vi "DataLog Tag and Meta Live_srv.vi"(0 "initial?":bool, 5 "read indices in":i32[](array[numeric]), 7 "certificate":string, 11 "base tag":string) -> (6 "read indices out":i32[](array[numeric]), 8 "points per tag":cluster{T1[]}[](array[cluster]) {"?"."value" format="%.3e"; "?"."time" format="%<%H:%M:%S%2u\n%Y/%m/%d>T"}, 10 "time":dbl format="%<%H:%M:%S%2u\n%Y/%m/%d>T", 15 "error out":errorcluster)   [LabVIEW 2012]
doc: "Reads all (when initial is true) or newer (when initial is false) data points from the in-memory buffers of a subset of tags. The read indices beyond the last read point are also returned. This allows a remote exhaustive read of multiple tags using a single VI server call thereby minimizing network load and latency."
uses:
  typedefs/clusters/t_DataLog Point.ctl
  typedefs/t_DataLog Tag Meta Tags Methods.ctl
  typedefs/t_DataLog Tag Hash Methods.ctl
  clientsrv/typedefs/t_ClientSrv Access Levels.ctl
  typedefs/t_DataLog Tag Buffers Methods.ctl
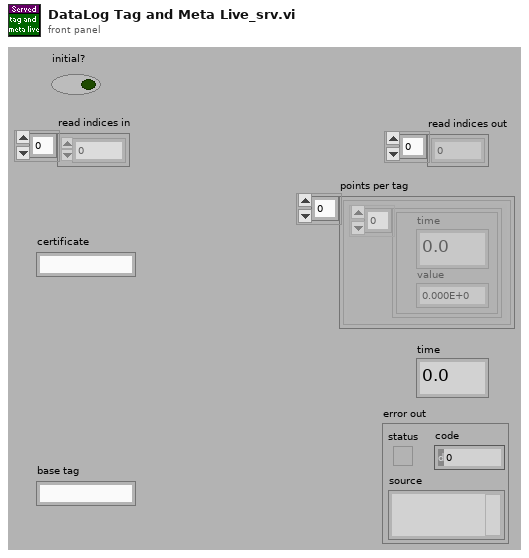
[diagram p1: front panel]
types:
  T1 = typedef "t_DataLog Point.ctl" = cluster{"time":dbl, "value":dbl}
  T2 = typedef "t_ClientSrv Access Levels.ctl" = enum16{"observer", "operator", "local"}
  T3 = typedef "t_DataLog Tag Hash Methods.ctl" = enum16{"initialize", "add tag", "index tag", "lookup", "#tags", "cleanup", "write recovery", "read recovery", "delete recovery"}
  T4 = typedef "t_DataLog Tag Meta Tags Methods.ctl" = enum16{"initialize", "apply and write", "get exceeded", "get metas", "cleanup"}
  T5 = typedef "t_DataLog Tag Buffers Methods.ctl" = enum16{"initialize", "inert", "write", "read", "read oldest", "read last", "cleanup"}
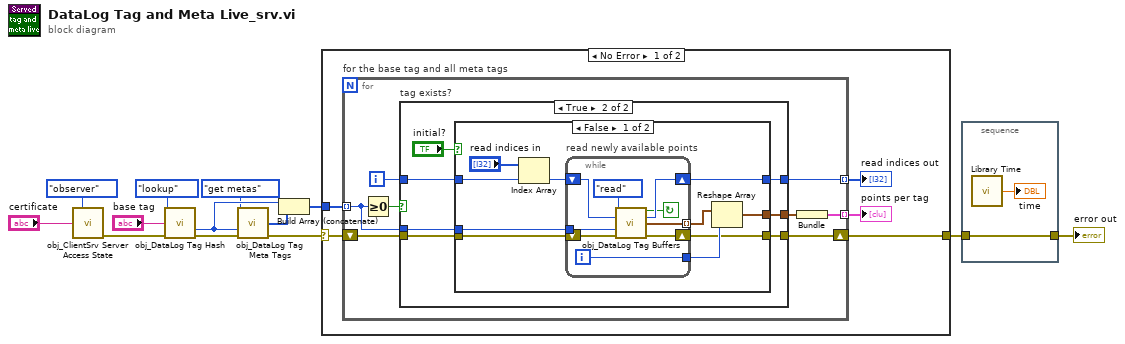
[diagram p0: block diagram]
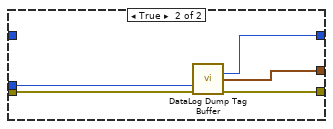
[diagram p3: hidden frame]
diagram:
  n1 = call "obj_ClientSrv Server Access State.vi"("access level"=t_ClientSrv_Access_Levels."observer", "certificate in"="certificate") -> ("error out"=w3:errorcluster)  [unwired: 11 in, 2 out]
  n2 = call "obj_DataLog Tag Hash.vi"("method"=t_DataLog_Tag_Hash_Methods."lookup", "tag in"="base tag", "error in (no error)"=w3) -> ("tag index out"=w12:i32, "error out"=w8:errorcluster)  [unwired: 9 in, 2 out]
  n3 = call "obj_DataLog Tag Meta Tags.vi"("method"=t_DataLog_Tag_Meta_Tags_Methods."get metas", "tag index in"=w12, "error in (no error)"=w8) -> ("meta tag indices (-1 if none)"=w13:i32[], "error out"=w6:errorcluster)  [unwired: 8 in, 3 out]
  n4 = Build Array (concatenate)(w12, w13) -> (w7:i32[])
  n5 = case shown="No Error" w6 {
    selector: w6 -> [w17 w59]
    tunnel: w7 -> [w18 _]
    tunnel: [w16 w59] -> w5
    frame No Error {
      n6 = for "for the base tag and all meta tags" {
        tunnel: w18 -> [w25] mode=indexing
        shift-right: [w23] -> w16
        shift-left: w17 -> [w24]
        tunnel: [w21] -> w15 mode=indexing
        tunnel: [w20] -> w14 mode=indexing
        i -> [w19]
        n7 = Greater Or Equal To 0?(x=w25) -> (x >= 0?=w26:bool)
        n8 = case "tag exists?" shown="True" w26 {
          tunnel: w25 -> [_ w29]
          tunnel: w24 -> [w27 w33]
          tunnel: [w27 w32] -> w23
          tunnel: [_ w31] -> w22
          tunnel: [_ w30] -> w20
          tunnel: w19 -> [_ w28]
          frame False {
          }
          frame True {
            n9 = case shown="False" "initial?" {
              tunnel: w33 -> [w44 w58]
              tunnel: [w38 w57] -> w32
              tunnel: [w40 w56] -> w31
              tunnel: [w42 w54] -> w30
              tunnel: w29 -> [w43 w55]
              tunnel: w28 -> [w35 _]
              frame False {
                n10 = Index Array(array="read indices in", index=w35) -> (element=w37:i32)
                n11 = while "read newly available points" {
                  shift-right: [w52] -> w38
                  shift-left: w44 -> [w53]
                  tunnel: w43 -> [w50]
                  shift-right: [w48] -> w42
                  shift-left: w37 -> [w49]
                  tunnel: [w46] -> w41 mode=indexing
                  tunnel: [w45] -> w39
                  i -> [w45]
                  stop <- w47 continue-if-true
                  n12 = call "obj_DataLog Tag Buffers.vi"("method"=t_DataLog_Tag_Buffers_Methods."read", "read index in"=w49, "tag index"=w50, "error in (no error)"=w53) -> ("available?"=w47:bool, "read index out"=w48:i32, "point out"=w46:T1, "error out"=w52:errorcluster)  [unwired: 7 in, 1 out]
                }
                n13 = Reshape Array(w41, w39) -> (w40:T1[])
              }
              frame True {
                n14 = call "DataLog Dump Tag Buffer.vi"("tag index"=w55, "error in (no error)"=w58) -> ("read index"=w54:i32, "points"=w56:T1[], "error out"=w57:errorcluster)  [unwired: 10 in, 1 out]
              }
            }
          }
        }
        n15 = Bundle("points"=w22) -> (w21:cluster{"points":T1[]})  [unwired: 1 in]
      }
      "points per tag" <- w15
      "read indices out" <- w14
    }
    frame Error {
    }
  }
  n16 = stacked-sequence {
    tunnel: w5 -> [w60]
    tunnel: [w60] -> w4
    frame #0 {
      n17 = call "Library Time.vi"() -> ("time"=→"time":dbl)  [unwired: 1 in]
    }
  }
  "error out" <- w4
